vi "ACK.vi"(8 "error in (no error)":errorcluster, 11 "Instrument in":refnum<class "Instrument.lvclass">) -> (0 "error out":errorcluster, 2 "ACK":string, 3 "Instrument out":refnum<class "Instrument.lvclass">)   [LabVIEW 2019, in "Instrument.lvlib" / "Instrument.lvclass"]
doc: "Send \"ACK\" command to remote Instrument to test connectivity."
uses:
  Instrument.lvclass
  Typedefs/Instrument.Commands--Enum.ctl
  f7bd5210-6898-44d9-a8a8-036b7bc7be21.vi
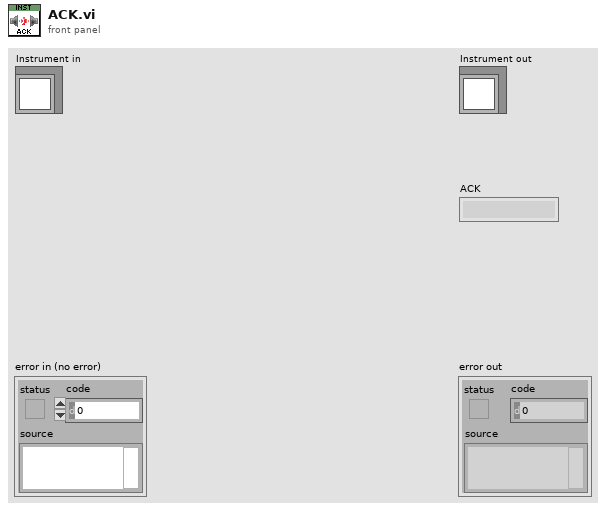
[diagram p1: front panel]
types:
  T1 = typedef "Instrument.lvlib/Instrument.lvclass/Instrument.Commands--Enum.ctl" = enum16{"ACK", "HELP", "IDN", "getAll", "getAllData"}
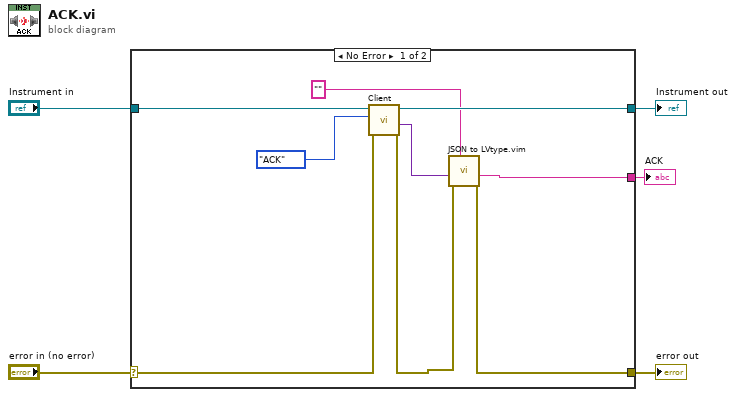
[diagram p0: block diagram]
diagram:
  n1 = case shown="No Error" "error in (no error)" {
    selector: "error in (no error)" -> [w12 w16]
    tunnel: [w7 w16] -> w4
    tunnel: [w14 w15] -> w2
    tunnel: "Instrument in" -> [w13 w15]
    tunnel: [w6 _] -> w1
    frame No Error {
      n2 = call-dynamic "Client.vi"("error in (no error)"=w12, "Command in"=Instrument.Commands--Enum."ACK" ("Commands"), "Instrument in"=w13) -> ("error out"=w8:errorcluster, "Data out"=w9:variant, "Instrument out"=w14:refnum<class "Instrument.lvclass">)  [unwired: 5 in, 1 out]
      n3 = call "JSON to LVtype.vim"("type"="" ("Commands"), "error in (no error)"=w8, "JSON Data in"=w9) -> ("error out"=w7:errorcluster, "Data out"=w6:string)  [unwired: 7 in]
    }
    frame Error {
    }
  }
  "error out" <- w4
  "Instrument out" <- w2
  "ACK" <- w1
